vi "Generate Bitfile Path.vi"() -> (0 "Bitfile Path":path)   [LabVIEW 2019]
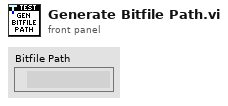
[diagram p1: front panel]
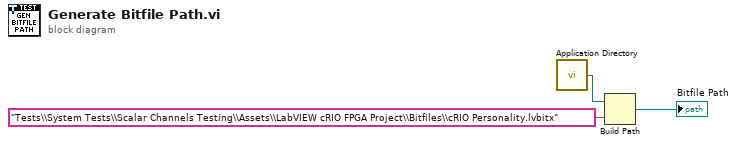
[diagram p0: block diagram]
diagram:
  n1 = call <vilib>:"Application Directory.vi"() -> ("Application Directory"=w2:path)
  n2 = Build Path(base path=w2, name or relative path="Tests\\System Tests\\Scalar Channels Testing\\Assets\\LabVIEW cRIO FPGA Project\\Bitfiles\\cRIO Personality.lvbitx") -> (appended path=→"Bitfile Path":path)
